vi "setra_2301_002PD_2F2D.vi"(1 "Output Unit":string(combo)="Pa", 2 "Source":dbl[](array[numeric]) format="%#_13g") -> (0 "Target":dbl[](array[numeric]) format="%#_13g")   [LabVIEW 2017, in "sensor_translation.lvlib"]
uses:
  sensor_translation.lvlib
  pressure_unit_converter.vi
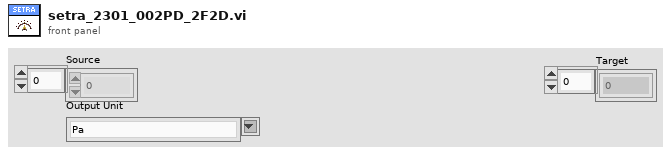
[diagram p1: front panel]
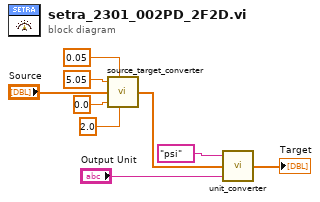
[diagram p0: block diagram]
diagram:
  n1 = call "source_target_converter.vi"("Source High"=5.05, "Source Low"=0.05, "Source"="Source", "Target Low"=0.0 ("Target High"), "Target High"=2.0 ("Target Low")) -> ("Target"=w4:dbl[])
  n2 = call-poly "unit_converter.vi"("Output Unit"="Output Unit", "Input"=w4, "Input Unit"="psi") -> ("Output"=→"Target":dbl[])
